vi "Configure Burst.vi"(4 "Burst Delay  (0.0 ns)":dbl format="%#.6g", 6 "Burst Count (5)":i32=5, 7 "Enable Burst (T: Enable)":bool=TRUE, 8 "error in (no error)":errorcluster, 9 "Burst Mode (0: Triggered)":u16(ring) items=["Triggered", "Gated"], 10 "Channel (0: Channel 1)":u16(ring) items=["Channel 1", "Channel 2"], 11 "VISA resource name":refnum<visa-resource-name>) -> (0 "error out":errorcluster, 3 "VISA resource name out":refnum<visa-resource-name>)   [LabVIEW 2018, in "AWG.lvlib" / "Tektronix AFG 3000 Series.lvlib"]
doc: "Allows and configures burst modulation. Configures the function generator to output a waveform with specified number of cycles, called burst. The carrier waveform shape and parameters are set by Configure Standard Waveform."
uses:
  Tektronix AFG 3000 Series.lvlib
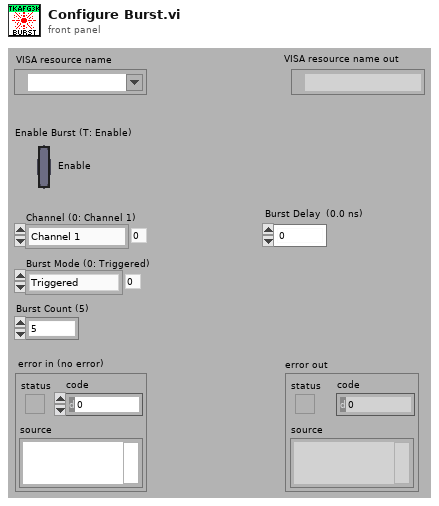
[diagram p1: front panel]
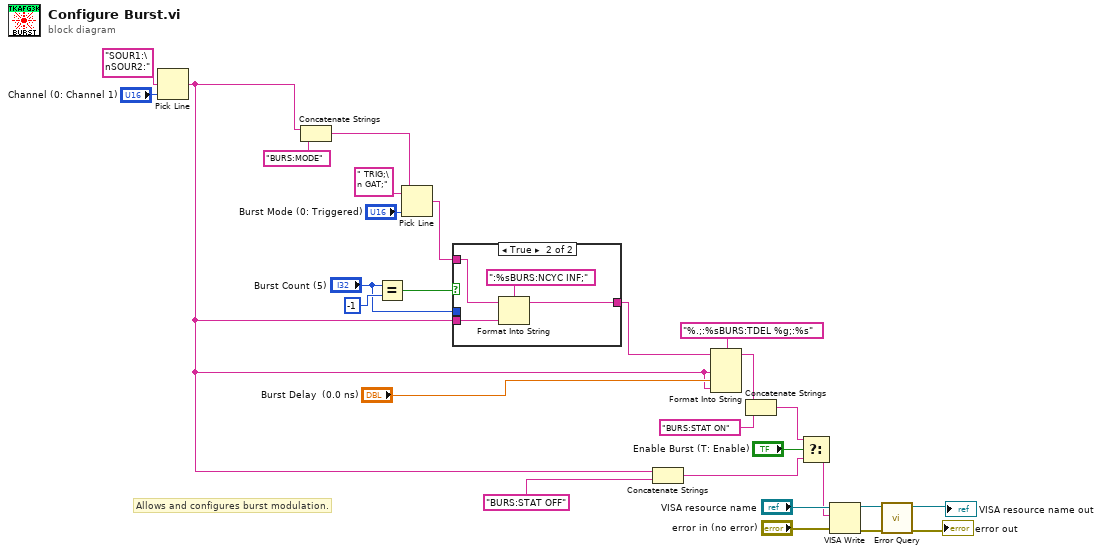
[diagram p0: block diagram]
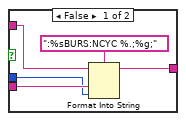
[diagram p2: hidden frame]
diagram:
  # "Allows and configures burst modulation."
  n1 = Pick Line(multi-line string="SOUR1:\nSOUR2:" ("string (\"\")"), line index="Channel (0: Channel 1)") -> (output string=w4:string)  [unwired: 1 in]
  n2 = Concatenate Strings(w4, "BURS:MODE" ("format string")) -> (w12:string)
  n3 = Equal?(x="Burst Count (5)", y=-1) -> (x = y?=w5:bool)
  n4 = Pick Line(string ("")=w12, multi-line string=" TRIG;\n GAT;" ("string (\"\")"), line index="Burst Mode (0: Triggered)") -> (output string=w3:string)
  n5 = case shown="True" w5 {
    tunnel: w4 -> [w32 w35]
    tunnel: w3 -> [w30 w34]
    tunnel: "Burst Count (5)" -> [w29 _]
    tunnel: [w28 w33] -> w1
    frame False {
      n6 = Format Into String(format string=":%sBURS:NCYC %.;%g;", initial string=w30, w32, w29) -> (resulting string=w28:string)  [unwired: 1 in, 1 out]
    }
    frame True {
      n7 = Format Into String(format string=":%sBURS:NCYC INF;", initial string=w34, w35) -> (resulting string=w33:string)  [unwired: 1 in, 1 out]
    }
  }
  n8 = Concatenate Strings(w4, "BURS:STAT OFF" ("string")) -> (w11:string)
  n9 = Format Into String(format string="%.;:%sBURS:TDEL %g;:%s", initial string=w1, w4, "Burst Delay  (0.0 ns)", w4) -> (resulting string=w7:string)  [unwired: 1 in, 1 out]
  n10 = Concatenate Strings(w7, "BURS:STAT ON" ("string")) -> (w18:string)
  n11 = Select(t=w18, s="Enable Burst (T: Enable)", f=w11) -> (s? t:f=w16:string)
  n12 = VISA Write(VISA resource name="VISA resource name", write buffer=w16, error in (no error)="error in (no error)") -> (VISA resource name out=w25:refnum<visa-resource-name>, error out=w24:errorcluster)  [unwired: 1 out]
  n13 = call "Error Query.vi"("error in (no error)"=w24, "VISA resource name"=w25) -> ("error out"=→"error out":errorcluster, "VISA resource name out"=→"VISA resource name out":refnum<visa-resource-name>)  [unwired: 6 in, 2 out]
